vi "Process Packet.vi"(8 "error in (no error)":errorcluster, 10 "Incoming Packet":refnum<class "ControlPacket.lvclass">, 11 "Session in":refnum<class "Session.lvclass">) -> (0 "error out":errorcluster, 3 "Session out":refnum<class "Session.lvclass">)   [LabVIEW 2013, in "MQTT Base.lvlib" / "Session.lvclass"]
uses:
  Session.lvclass
  <vilib>/LabVIEW Open Source Project/MQTT Control Packets/Control Packets/ControlPacket/ControlPacket.lvclass
  Base Class/Request -- cluster.ctl
  Base Class/Response -- cluster.ctl
  Session.lvclass/Session.ctl
  <vilib>/LabVIEW Open Source Project/MQTT Control Packets/Control Packets/ControlPacket/ControlPacket.lvclass/ControlPacket.ctl
  Read SessionState.vi
  Base Class/MQTT_Base.lvclass
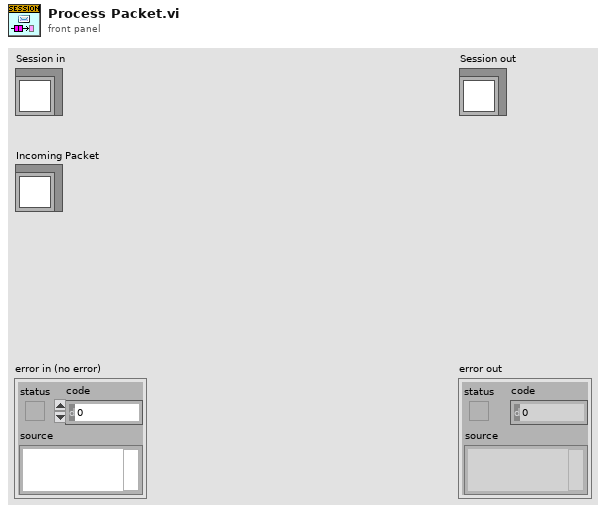
[diagram p1: front panel]
types:
  T1 = typedef "MQTT Base.lvlib/MQTT_Base.lvclass/Request -- cluster.ctl" = cluster{"Packet":refnum<class "ControlPacket.lvclass">, "SessionMailbox":refnum<queue>}
  T2 = typedef "MQTT Base.lvlib/MQTT_Base.lvclass/Response -- cluster.ctl" = cluster{"Packet":refnum<class "ControlPacket.lvclass">, "Protocol Error":errorcluster, "disconnect session":bool, "[ACK]":refnum<notifier>[]}
  T3 = typedef "MQTT Base.lvlib/Session.lvclass/Pending ACKs -- cluster.ctl" = cluster{"Message":refnum<class "ControlPacket.lvclass">, "[ACK]":refnum<notifier>[], "Packet Identifier":u16}
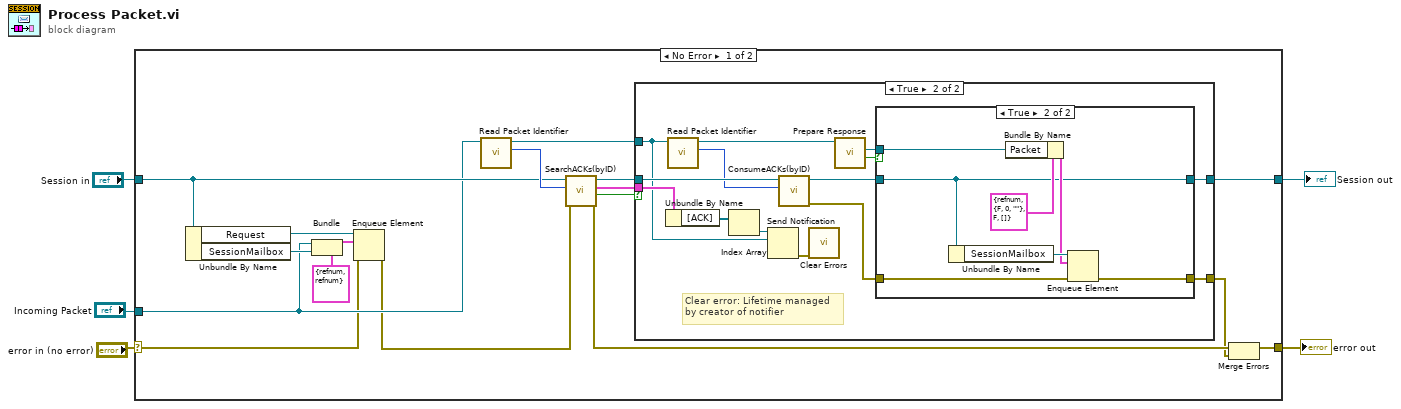
[diagram p0: block diagram]
diagram:
  n1 = case shown="No Error" "error in (no error)" {
    selector: "error in (no error)" -> [w7 w48]
    tunnel: [w19 w48] -> w1
    tunnel: [w15 w47] -> w2
    tunnel: "Session in" -> [w9 w47]
    tunnel: "Incoming Packet" -> [w8 _]
    frame No Error {
      n2 = Unbundle By Name(w9) -> ("Request"=w10:refnum<queue>, "SessionMailbox"=w11:refnum<queue>)
      n3 = Bundle(cluster=T1 {"Packet"=refnum, "SessionMailbox"=refnum} ("Request"), "Packet"=w8, "SessionMailbox"=w11) -> (w12:T1)
      n4 = Enqueue Element(queue=w10, element=w12, error in (no error)=w7) -> (error out=w6:errorcluster)  [unwired: 1 in, 2 out]
      n5 = call <vilib>:"Read Packet Identifier.vi"("ControlPacket in"=w8) -> ("Packet Identifier"=w18:u16, "ControlPacket out"=w17:refnum<class "ControlPacket.lvclass">)  [unwired: 9 in]
      n6 = call "SearchACKs(byID).vi"("error in (no error)"=w6, "Packet Identifier"=w18, "Session in"=w9) -> ("error out"=w16:errorcluster, "found?"=w22:bool, "Pending ACK"=w21:T3, "Session out"=w20:refnum<class "Session.lvclass">)  [unwired: 5 in]
      n7 = case shown="True" w22 {
        tunnel: w21 -> [_ w34]
        tunnel: w20 -> [w23 w33]
        tunnel: [w23 w32] -> w15
        tunnel: w17 -> [_ w31]
        tunnel: [_ w29] -> w14
        frame False {
        }
        frame True {
          # "Clear error: Lifetime managed\nby creator of notifier"
          n8 = Unbundle By Name(w34) -> ("[ACK]"=w37:refnum<notifier>[])
          n9 = call <vilib>:"Read Packet Identifier.vi"("ControlPacket in"=w31) -> ("Packet Identifier"=w26:u16, "ControlPacket out"=w30:refnum<class "ControlPacket.lvclass">)  [unwired: 9 in]
          n10 = Index Array(array=w37) -> (element=w36:refnum<notifier>)  [unwired: 1 in]
          n11 = Send Notification(notification=w31, notifier=w36) -> (error out=w35:errorcluster)  [unwired: 1 in, 1 out]
          n12 = call "ConsumeACKs(byID).vi"("Packet Identifier"=w26, "Session in"=w33) -> ("error out"=w24:errorcluster, "Session out"=w25:refnum<class "Session.lvclass">)  [unwired: 8 in]
          n13 = call <vilib>:"Clear Errors.vi"("error in (no error)"=w35) -> ()  [unwired: 6 in, 1 out]
          n14 = call-dynamic "Prepare Response.vi"("ControlPacket in"=w30) -> ("response prepared?"=w28:bool, "ControlPacket response"=w27:refnum<class "ControlPacket.lvclass">)  [unwired: 7 in, 2 out]
          n15 = case shown="True" w28 {
            tunnel: w25 -> [w39 w40]
            tunnel: [w38 w43] -> w29
            tunnel: [w39 w40] -> w32
            tunnel: w27 -> [_ w42]
            tunnel: w24 -> [w38 w41]
            frame False {
            }
            frame True {
              n16 = Unbundle By Name(w40) -> ("SessionMailbox"=w46:refnum<queue>)
              n17 = Bundle By Name(cluster=T2 {"Packet"=refnum, "Protocol Error"={"status"=FALSE, "code"=0, "source"=""}, "disconnect session"=FALSE, "[ACK]"=[]} ("element"), "Packet"=w42) -> (w44:T2)
              n18 = Enqueue Element(queue=w46, element=w44, error in (no error)=w41) -> (error out=w43:errorcluster)  [unwired: 1 in, 2 out]
            }
          }
        }
      }
      n19 = Merge Errors(w16, w14) -> (w19:errorcluster)
    }
    frame Error {
    }
  }
  "error out" <- w1
  "Session out" <- w2
